vi "Read LogicOuts.vi"(8 "error in (no error)":errorcluster, 11 "VacuumLines in":refnum<class "VacuumLines.lvclass">) -> (0 "error out":errorcluster, 2 "LogicOut Statuses":bool[](array[boolean]), 3 "VacuumLines out":refnum<class "VacuumLines.lvclass">)   [LabVIEW 2016, in "Hardware.lvlib" / "VacuumLine.lvlib" / "VacuumLines.lvclass"]
uses:
  <userlib>/Common Components/Hardware/Abstract System/VacuumLine/VacuumLines/VacuumLines.lvclass
  <userlib>/Common Components/Hardware/Abstract System/VacuumLine/VacuumLines/VacuumLines.lvclass/VacuumLines.ctl
  <userlib>/Common Components/Hardware/Abstract System/VacuumLine/VacuumLine/VacuumLine.lvclass/VacuumLine.ctl
  <userlib>/Common Components/Hardware/Abstract System/VacuumLine/VacuumLine/Read Motor disconnected.vi
  <userlib>/Common Components/Hardware/LogicIO/LogicIO/Get Logic Status (single).vi
  <userlib>/Common Components/Hardware/LogicIO/LogicIO/LogicIO.lvclass
  <userlib>/Common Components/Hardware/Abstract System/VacuumLine/VacuumLine/VacuumLine.lvclass
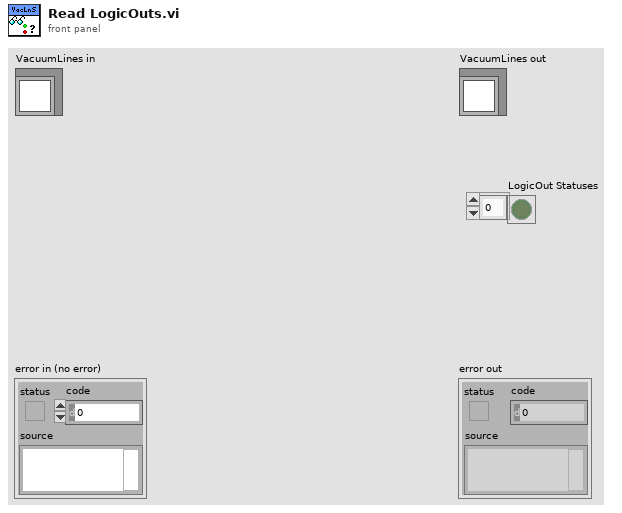
[diagram p1: front panel]
types:
  T1 = typedef "Hardware.lvlib/VacuumLine.lvlib/VacuumLines.lvclass/LogicOut.ctl" = cluster{"Label":string, "LogicIO Module":string, "Pin#":u8}
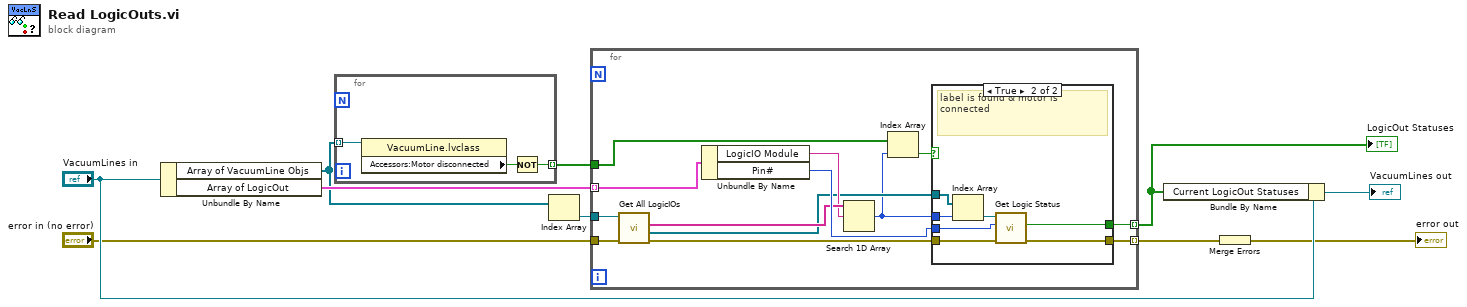
[diagram p0: block diagram]
diagram:
  n1 = Unbundle By Name("VacuumLines in") -> ("Array of VacuumLine Objs"=w2:refnum<class "VacuumLine.lvclass">[], "Array of LogicOut"=w9:T1[])
  n2 = for {
    tunnel: w2 -> [w13] mode=indexing
    tunnel: [w11] -> w1 mode=indexing
    n3 = property class="VacuumLine.lvclass"(reference=w13) -> ("Accessors:Motor disconnected"=w12:bool)  [unwired: 1 in, 2 out]
    n4 = Not(x=w12) -> (.not. x?=w11:bool)
  }
  n5 = Index Array(array=w2) -> (element=w8:refnum<class "VacuumLine.lvclass">)  [unwired: 1 in]
  n6 = for {
    tunnel: w9 -> [w26] mode=indexing
    tunnel: w8 -> [w22]
    tunnel: [w24] -> w4 mode=indexing
    tunnel: "error in (no error)" -> [w15]
    tunnel: [w23] -> w6 mode=indexing
    tunnel: w1 -> [w19]
    n7 = call <userlib>:"Get All LogicIOs.vi"("error in (no error)"=w15, "VacuumLine in"=w22) -> ("error out"=w14:errorcluster, "LogicIOs"=w17:refnum<class "LogicIO.lvclass">[], "labels"=w21:string[])  [unwired: 6 in, 1 out]
    n8 = Unbundle By Name(w26) -> ("LogicIO Module"=w20:string, "Pin#"=w25:u8)
    n9 = Search 1D Array(1D array=w21, element=w20) -> (index of element=w16:i32)  [unwired: 1 in]
    n10 = Index Array(array=w19, index=w16) -> (element=w18:bool)
    n11 = case shown="True" w18 {
      tunnel: w25 -> [_ w34]
      tunnel: [_ w33] -> w24
      tunnel: w14 -> [w27 w32]
      tunnel: [w27 w31] -> w23
      tunnel: w17 -> [_ w30]
      tunnel: w16 -> [_ w29]
      frame False {
      }
      frame True {
        # "label is found & motor is connected"
        n12 = Index Array(array=w30, index=w29) -> (element=w28:refnum<class "LogicIO.lvclass">)
        n13 = call-poly <userlib>:"Get Logic Status.vi"("error in (no error)"=w32, "Pin # (1-based)"=w34, "LogicIO in"=w28) -> ("error out"=w31:errorcluster, "logic status"=w33:bool)  [unwired: 6 in, 1 out]
      }
    }
  }
  "LogicOut Statuses" <- w4
  n14 = Bundle By Name(cluster="VacuumLines in", "Current LogicOut Statuses"=w4) -> (→"VacuumLines out":refnum<class "VacuumLines.lvclass">)
  n15 = Merge Errors(w6) -> (→"error out":errorcluster)
